vi "FipsAdjacent.vi"() -> (11 "Fips":i32[](array[numeric]))   [LabVIEW 2017] (continued)
IL\"\t17151\n\"Pope County, IL\"\t17151\t\"Saline County, IL\"\t17165\n\"Pope County, IL\"\t17151\t\"Williamson County, IL\"\t17199\n\"Pope County, IL\"\t17151\t\"Livingston County, KY\"\t21139\n\"Pulaski County, IL\"\t17153\t\"Alexander County, IL\"\t17003\n\"Pulaski County, IL\"\t17153\t\"Johnson County, IL\"\t17087\n\"Pulaski County, IL\"\t17153\t\"Massac County, IL\"\t17127\n\"Pulaski County, IL\"\t17153\t\"Pulaski County, IL\"\t17153\n\"Pulaski County, IL\"\t17153\t\"Union County, IL\"\t17181\n\"Pulaski County, IL\"\t17153\t\"Ballard County, KY\"\t21007\n\"Pulaski County, IL\"\t17153\t\"McCracken County, KY\"\t21145\n\"Putnam County, IL\"\t17155\t\"Bureau County, IL\"\t17011\n\"Putnam County, IL\"\t17155\t\"LaSalle County, IL\"\t17099\n\"Putnam County, IL\"\t17155\t\"Marshall County, IL\"\t17123\n\"Putnam County, IL\"\t17155\t\"Putnam County, IL\"\t17155\n\"Randolph County, IL\"\t17157\t\"Jackson County, IL\"\t17077\n\"Randolph County, IL\"\t17157\t\"Monroe County, IL\"\t17133\n\"Randolph County, IL\"\t17157\t\"Perry County, IL\"\t17145\n\"Randolph County, IL\"\t17157\t\"Randolph County, IL\"\t17157\n\"Randolph County, IL\"\t17157\t\"St. Clair County, IL\"\t17163\n\"Randolph County, IL\"\t17157\t\"Washington County, IL\"\t17189\n\"Randolph County, IL\"\t17157\t\"Perry County, MO\"\t29157\n\"Randolph County, IL\"\t17157\t\"Ste. Genevieve County, MO\"\t29186\n\"Richland County, IL\"\t17159\t\"Clay County, IL\"\t17025\n\"Richland County, IL\"\t17159\t\"Crawford County, IL\"\t17033\n\"Richland County, IL\"\t17159\t\"Edwards County, IL\"\t17047\n\"Richland County, IL\"\t17159\t\"Jasper County, IL\"\t17079\n\"Richland County, IL\"\t17159\t\"Lawrence County, IL\"\t17101\n\"Richland County, IL\"\t17159\t\"Richland County, IL\"\t17159\n\"Richland County, IL\"\t17159\t\"Wabash County, IL\"\t17185\n\"Richland County, IL\"\t17159\t\"Wayne County, IL\"\t17191\n\"Rock Island County, IL\"\t17161\t\"Henry County, IL\"\t17073\n\"Rock Island County, IL\"\t17161\t\"Mercer County, IL\"\t17131\n\"Rock Island County, IL\"\t17161\t\"Rock Island County, IL\"\t17161\n\"Rock Island County, IL\"\t17161\t\"Whiteside County, IL\"\t17195\n\"Rock Island County, IL\"\t17161\t\"Clinton County, IA\"\t19045\n\"Rock Island County, IL\"\t17161\t\"Louisa County, IA\"\t19115\n\"Rock Island County, IL\"\t17161\t\"Muscatine County, IA\"\t19139\n\"Rock Island County, IL\"\t17161\t\"Scott County, IA\"\t19163\n\"St. Clair County, IL\"\t17163\t\"Clinton County, IL\"\t17027\n\"St. Clair County, IL\"\t17163\t\"Madison County, IL\"\t17119\n\"St. Clair County, IL\"\t17163\t\"Monroe County, IL\"\t17133\n\"St. Clair County, IL\"\t17163\t\"Randolph County, IL\"\t17157\n\"St. Clair County, IL\"\t17163\t\"St. Clair County, IL\"\t17163\n\"St. Clair County, IL\"\t17163\t\"Washington County, IL\"\t17189\n\"St. Clair County, IL\"\t17163\t\"St. Louis County, MO\"\t29189\n\"St. Clair County, IL\"\t17163\t\"St. Louis city, MO\"\t29510\n\"Saline County, IL\"\t17165\t\"Franklin County, IL\"\t17055\n\"Saline County, IL\"\t17165\t\"Gallatin County, IL\"\t17059\n\"Saline County, IL\"\t17165\t\"Hamilton County, IL\"\t17065\n\"Saline County, IL\"\t17165\t\"Hardin County, IL\"\t17069\n\"Saline County, IL\"\t17165\t\"Johnson County, IL\"\t17087\n\"Saline County, IL\"\t17165\t\"Pope County, IL\"\t17151\n\"Saline County, IL\"\t17165\t\"Saline County, IL\"\t17165\n\"Saline County, IL\"\t17165\t\"Williamson County, IL\"\t17199\n\"Sangamon County, IL\"\t17167\t\"Cass County, IL\"\t17017\n\"Sangamon County, IL\"\t17167\t\"Christian County, IL\"\t17021\n\"Sangamon County, IL\"\t17167\t\"Logan County, IL\"\t17107\n\"Sangamon County, IL\"\t17167\t\"Macon County, IL\"\t17115\n\"Sangamon County, IL\"\t17167\t\"Macoupin County, IL\"\t17117\n\"Sangamon County, IL\"\t17167\t\"Menard County, IL\"\t17129\n\"Sangamon County, IL\"\t17167\t\"Montgomery County, IL\"\t17135\n\"Sangamon County, IL\"\t17167\t\"Morgan County, IL\"\t17137\n\"Sangamon County, IL\"\t17167\t\"Sangamon County, IL\"\t17167\n\"Schuyler County, IL\"\t17169\t\"Adams County, IL\"\t17001\n\"Schuyler County, IL\"\t17169\t\"Brown County, IL\"\t17009\n\"Schuyler County, IL\"\t17169\t\"Cass County, IL\"\t17017\n\"Schuyler County, IL\"\t17169\t\"Fulton County, IL\"\t17057\n\"Schuyler County, IL\"\t17169\t\"Hancock County, IL\"\t17067\n\"Schuyler County, IL\"\t17169\t\"McDonough County, IL\"\t17109\n\"Schuyler County, IL\"\t17169\t\"Mason County, IL\"\t17125\n\"Schuyler County, IL\"\t17169\t\"Schuyler County, IL\"\t17169\n\"Scott County, IL\"\t17171\t\"Greene County, IL\"\t17061\n\"Scott County, IL\"\t17171\t\"Morgan County, IL\"\t17137\n\"Scott County, IL\"\t17171\t\"Pike County, IL\"\t17149\n\"Scott County, IL\"\t17171\t\"Scott County, IL\"\t17171\n\"Shelby County, IL\"\t17173\t\"Christian County, IL\"\t17021\n\"Shelby County, IL\"\t17173\t\"Coles County, IL\"\t17029\n\"Shelby County, IL\"\t17173\t\"Cumberland County, IL\"\t17035\n\"Shelby County, IL\"\t17173\t\"Effingham County, IL\"\t17049\n\"Shelby County, IL\"\t17173\t\"Fayette County, IL\"\t17051\n\"Shelby County, IL\"\t17173\t\"Macon County, IL\"\t17115\n\"Shelby County, IL\"\t17173\t\"Montgomery County, IL\"\t17135\n\"Shelby County, IL\"\t17173\t\"Moultrie County, IL\"\t17139\n\"Shelby County, IL\"\t17173\t\"Shelby County, IL\"\t17173\n\"Stark County, IL\"\t17175\t\"Bureau County, IL\"\t17011\n\"Stark County, IL\"\t17175\t\"Henry County, IL\"\t17073\n\"Stark County, IL\"\t17175\t\"Knox County, IL\"\t17095\n\"Stark County, IL\"\t17175\t\"Marshall County, IL\"\t17123\n\"Stark County, IL\"\t17175\t\"Peoria County, IL\"\t17143\n\"Stark County, IL\"\t17175\t\"Stark County, IL\"\t17175\n\"Stephenson County, IL\"\t17177\t\"Carroll County, IL\"\t17015\n\"Stephenson County, IL\"\t17177\t\"Jo Daviess County, IL\"\t17085\n\"Stephenson County, IL\"\t17177\t\"Ogle County, IL\"\t17141\n\"Stephenson County, IL\"\t17177\t\"Stephenson County, IL\"\t17177\n\"Stephenson County, IL\"\t17177\t\"Winnebago County, IL\"\t17201\n\"Stephenson County, IL\"\t17177\t\"Green County, WI\"\t55045\n\"Stephenson County, IL\"\t17177\t\"Lafayette County, WI\"\t55065\n\"Tazewell County, IL\"\t17179\t\"Fulton County, IL\"\t17057\n\"Tazewell County, IL\"\t17179\t\"Logan County, IL\"\t17107\n\"Tazewell County, IL\"\t17179\t\"McLean County, IL\"\t17113\n\"Tazewell County, IL\"\t17179\t\"Mason County, IL\"\t17125\n\"Tazewell County, IL\"\t17179\t\"Peoria County, IL\"\t17143\n\"Tazewell County, IL\"\t17179\t\"Tazewell County, IL\"\t17179\n\"Tazewell County, IL\"\t17179\t\"Woodford County, IL\"\t17203\n\"Union County, IL\"\t17181\t\"Alexander County, IL\"\t17003\n\"Union County, IL\"\t17181\t\"Jackson County, IL\"\t17077\n\"Union County, IL\"\t17181\t\"Johnson County, IL\"\t17087\n\"Union County, IL\"\t17181\t\"Pulaski County, IL\"\t17153\n\"Union County, IL\"\t17181\t\"Union County, IL\"\t17181\n\"Union County, IL\"\t17181\t\"Williamson County, IL\"\t17199\n\"Union County, IL\"\t17181\t\"Cape Girardeau County, MO\"\t29031\n\"Union County, IL\"\t17181\t\"Perry County, MO\"\t29157\n\"Vermilion County, IL\"\t17183\t\"Champaign County, IL\"\t17019\n\"Vermilion County, IL\"\t17183\t\"Douglas County, IL\"\t17041\n\"Vermilion County, IL\"\t17183\t\"Edgar County, IL\"\t17045\n\"Vermilion County, IL\"\t17183\t\"Ford County, IL\"\t17053\n\"Vermilion County, IL\"\t17183\t\"Iroquois County, IL\"\t17075\n\"Vermilion County, IL\"\t17183\t\"Vermilion County, IL\"\t17183\n\"Vermilion County, IL\"\t17183\t\"Benton County, IN\"\t18007\n\"Vermilion County, IL\"\t17183\t\"Vermillion County, IN\"\t18165\n\"Vermilion County, IL\"\t17183\t\"Warren County, IN\"\t18171\n\"Wabash County, IL\"\t17185\t\"Edwards County, IL\"\t17047\n\"Wabash County, IL\"\t17185\t\"Lawrence County, IL\"\t17101\n\"Wabash County, IL\"\t17185\t\"Richland County, IL\"\t17159\n\"Wabash County, IL\"\t17185\t\"Wabash County, IL\"\t17185\n\"Wabash County, IL\"\t17185\t\"White County, IL\"\t17193\n\"Wabash County, IL\"\t17185\t\"Gibson County, IN\"\t18051\n\"Wabash County, IL\"\t17185\t\"Knox County, IN\"\t18083\n\"Warren County, IL\"\t17187\t\"Fulton County, IL\"\t17057\n\"Warren County, IL\"\t17187\t\"Henderson County, IL\"\t17071\n\"Warren County, IL\"\t17187\t\"Knox County, IL\"\t17095\n\"Warren County, IL\"\t17187\t\"McDonough County, IL\"\t17109\n\"Warren County, IL\"\t17187\t\"Mercer County, IL\"\t17131\n\"Warren County, IL\"\t17187\t\"Warren County, IL\"\t17187\n\"Washington County, IL\"\t17189\t\"Clinton County, IL\"\t17027\n\"Washington County, IL\"\t17189\t\"Jefferson County, IL\"\t17081\n\"Washington County, IL\"\t17189\t\"Marion County, IL\"\t17121\n\"Washington County, IL\"\t17189\t\"Perry County, IL\"\t17145\n\"Washington County, IL\"\t17189\t\"Randolph County, IL\"\t17157\n\"Washington County, IL\"\t17189\t\"St. Clair County, IL\"\t17163\n\"Washington County, IL\"\t17189\t\"Washington County, IL\"\t17189\n\"Wayne County, IL\"\t17191\t\"Clay County, IL\"\t17025\n\"Wayne County, IL\"\t17191\t\"Edwards County, IL\"\t17047\n\"Wayne County, IL\"\t17191\t\"Hamilton County, IL\"\t17065\n\"Wayne County, IL\"\t17191\t\"Jefferson County, IL\"\t17081\n\"Wayne County, IL\"\t17191\t\"Marion County, IL\"\t17121\n\"Wayne County, IL\"\t17191\t\"Richland County, IL\"\t17159\n\"Wayne County, IL\"\t17191\t\"Wayne County, IL\"\t17191\n\"Wayne County, IL\"\t17191\t\"White County, IL\"\t17193\n\"White County, IL\"\t17193\t\"Edwards County, IL\"\t17047\n\"White County, IL\"\t17193\t\"Gallatin County, IL\"\t17059\n\"White County, IL\"\t17193\t\"Hamilton County, IL\"\t17065\n\"White County, IL\"\t17193\t\"Wabash County, IL\"\t17185\n\"White County, IL\"\t17193\t\"Wayne County, IL\"\t17191\n\"White County, IL\"\t17193\t\"White County, IL\"\t17193\n\"White County, IL\"\t17193\t\"Gibson County, IN\"\t18051\n\"White County, IL\"\t17193\t\"Posey County, IN\"\t18129\n\"Whiteside County, IL\"\t17195\t\"Bureau County, IL\"\t17011\n\"Whiteside County, IL\"\t17195\t\"Carroll County, IL\"\t17015\n\"Whiteside County, IL\"\t17195\t\"Henry County, IL\"\t17073\n\"Whiteside County, IL\"\t17195\t\"Lee County, IL\"\t17103\n\"Whiteside County, IL\"\t17195\t\"Ogle County, IL\"\t17141\n\"Whiteside County, IL\"\t17195\t\"Rock Island County, IL\"\t17161\n\"Whiteside County, IL\"\t17195\t\"Whiteside County, IL\"\t17195\n\"Whiteside County, IL\"\t17195\t\"Clinton County, IA\"\t19045\n\"Will County, IL\"\t17197\t\"Cook County, IL\"\t17031\n\"Will County, IL\"\t17197\t\"DuPage County, IL\"\t17043\n\"Will County, IL\"\t17197\t\"Grundy County, IL\"\t17063\n\"Will County, IL\"\t17197\t\"Kankakee County, IL\"\t17091\n\"Will County, IL\"\t17197\t\"Kendall County, IL\"\t17093\n\"Will County, IL\"\t17197\t\"Will County, IL\"\t17197\n\"Will County, IL\"\t17197\t\"Lake County, IN\"\t18089\n\"Williamson County, IL\"\t17199\t\"Franklin County, IL\"\t17055\n\"Williamson County, IL\"\t17199\t\"Jackson County, IL\"\t17077\n\"Williamson County, IL\"\t17199\t\"Johnson County, IL\"\t17087\n\"Williamson County, IL\"\t17199\t\"Pope County, IL\"\t17151\n\"Williamson County, IL\"\t17199\t\"Saline County, IL\"\t17165\n\"Williamson County, IL\"\t17199\t\"Union County, IL\"\t17181\n\"Williamson County, IL\"\t17199\t\"Williamson County, IL\"\t17199\n\"Winnebago County, IL\"\t17201\t\"Boone County, IL\"\t17007\n\"Winnebago County, IL\"\t17201\t\"DeKalb County, IL\"\t17037\n\"Winnebago County, IL\"\t17201\t\"Ogle County, IL\"\t17141\n\"Winnebago County, IL\"\t17201\t\"Stephenson County, IL\"\t17177\n\"Winnebago County, IL\"\t17201\t\"Winnebago County, IL\"\t17201\n\"Winnebago County, IL\"\t17201\t\"Green County, WI\"\t55045\n\"Winnebago County, IL\"\t17201\t\"Rock County, WI\"\t55105\n\"Woodford County, IL\"\t17203\t\"LaSalle County, IL\"\t17099\n\"Woodford County, IL\"\t17203\t\"Livingston County, IL\"\t17105\n\"Woodford County, IL\"\t17203\t\"McLean County, IL\"\t17113\n\"Woodford County, IL\"\t17203\t\"Marshall County, IL\"\t17123\n\"Woodford County, IL\"\t17203\t\"Peoria County, IL\"\t17143\n\"Woodford County, IL\"\t17203\t\"Tazewell County, IL\"\t17179\n\"Woodford County, IL\"\t17203\t\"Woodford County, IL\"\t17203\n\"Adams County, IN\"\t18001\t\"Adams County, IN\"\t18001\n\"Adams County, IN\"\t18001\t\"Allen County, IN\"\t18003\n\"Adams County, IN\"\t18001\t\"Jay County, IN\"\t18075\n\"Adams County, IN\"\t18001\t\"Wells County, IN\"\t18179\n\"Adams County, IN\"\t18001\t\"Mercer County, OH\"\t39107\n\"Adams County, IN\"\t18001\t\"Van Wert County, OH\"\t39161\n\"Allen County, IN\"\t18003\t\"Adams County, IN\"\t18001\n\"Allen County, IN\"\t18003\t\"Allen County, IN\"\t18003\n\"Allen County, IN\"\t18003\t\"DeKalb County, IN\"\t18033\n\"Allen County, IN\"\t18003\t\"Huntington County, IN\"\t18069\n\"Allen County, IN\"\t18003\t\"Noble County, IN\"\t18113\n\"Allen County, IN\"\t18003\t\"Wells County, IN\"\t18179\n\"Allen County, IN\"\t18003\t\"Whitley County, IN\"\t18183\n\"Allen County, IN\"\t18003\t\"Defiance County, OH\"\t39039\n\"Allen County, IN\"\t18003\t\"Paulding County, OH\"\t39125\n\"Allen County, IN\"\t18003\t\"Van Wert County, OH\"\t39161\n\"Bartholomew County, IN\"\t18005\t\"Bartholomew County, IN\"\t18005\n\"Bartholomew County, IN\"\t18005\t\"Brown County, IN\"\t18013\n\"Bartholomew County, IN\"\t18005\t\"Decatur County, IN\"\t18031\n\"Bartholomew County, IN\"\t18005\t\"Jackson County, IN\"\t18071\n\"Bartholomew County, IN\"\t18005\t\"Jennings County, IN\"\t18079\n\"Bartholomew County, IN\"\t18005\t\"Johnson County, IN\"\t18081\n\"Bartholomew County, IN\"\t18005\t\"Shelby County, IN\"\t18145\n\"Benton County, IN\"\t18007\t\"Iroquois County, IL\"\t17075\n\"Benton County, IN\"\t18007\t\"Vermilion County, IL\"\t17183\n\"Benton County, IN\"\t18007\t\"Benton County, IN\"\t18007\n\"Benton County, IN\"\t18007\t\"Jasper County, IN\"\t18073\n\"Benton County, IN\"\t18007\t\"Newton County, IN\"\t18111\n\"Benton County, IN\"\t18007\t\"Tippecanoe County, IN\"\t18157\n\"Benton County, IN\"\t18007\t\"Warren County, IN\"\t18171\n\"Benton County, IN\"\t18007\t\"White County, IN\"\t18181\n\"Blackford County, IN\"\t18009\t\"Blackford County, IN\"\t18009\n\"Blackford County, IN\"\t18009\t\"Delaware County, IN\"\t18035\n\"Blackford County, IN\"\t18009\t\"Grant County, IN\"\t18053\n\"Blackford County, IN\"\t18009\t\"Jay County, IN\"\t18075\n\"Blackford County, IN\"\t18009\t\"Wells County, IN\"\t18179\n\"Boone County, IN\"\t18011\t\"Boone County, IN\"\t18011\n\"Boone County, IN\"\t18011\t\"Clinton County, IN\"\t18023\n\"Boone County, IN\"\t18011\t\"Hamilton County, IN\"\t18057\n\"Boone County, IN\"\t18011\t\"Hendricks County, IN\"\t18063\n\"Boone County, IN\"\t18011\t\"Marion County, IN\"\t18097\n\"Boone County, IN\"\t18011\t\"Montgomery County, IN\"\t18107\n\"Brown County, IN\"\t18013\t\"Bartholomew County, IN\"\t18005\n\"Brown County, IN\"\t18013\t\"Brown County, IN\"\t18013\n\"Brown County, IN\"\t18013\t\"Jackson County, IN\"\t18071\n\"Brown County, IN\"\t18013\t\"Johnson County, IN\"\t18081\n\"Brown County, IN\"\t18013\t\"Monroe County, IN\"\t18105\n\"Brown County, IN\"\t18013\t\"Morgan County, IN\"\t18109\n\"Carroll County, IN\"\t18015\t\"Carroll County, IN\"\t18015\n\"Carroll County, IN\"\t18015\t\"Cass County, IN\"\t18017\n\"Carroll County, IN\"\t18015\t\"Clinton County, IN\"\t18023\n\"Carroll County, IN\"\t18015\t\"Howard County, IN\"\t18067\n\"Carroll County, IN\"\t18015\t\"Tippecanoe County, IN\"\t18157\n\"Carroll County, IN\"\t18015\t\"White County, IN\"\t18181\n\"Cass County, IN\"\t18017\t\"Carroll County, IN\"\t18015\n\"Cass County, IN\"\t18017\t\"Cass County, IN\"\t18017\n\"Cass County, IN\"\t18017\t\"Fulton County, IN\"\t18049\n\"Cass County, IN\"\t18017\t\"Howard County, IN\"\t18067\n\"Cass County, IN\"\t18017\t\"Miami County, IN\"\t18103\n\"Cass County, IN\"\t18017\t\"Pulaski County, IN\"\t18131\n\"Cass County, IN\"\t18017\t\"White County, IN\"\t18181\n\"Clark County, IN\"\t18019\t\"Clark County, IN\"\t18019\n\"Clark County, IN\"\t18019\t\"Floyd County, IN\"\t18043\n\"Clark County, IN\"\t18019\t\"Jefferson County, IN\"\t18077\n\"Clark County, IN\"\t18019\t\"Scott County, IN\"\t18143\n\"Clark County, IN\"\t18019\t\"Washington County, IN\"\t18175\n\"Clark County, IN\"\t18019\t\"Jefferson County, KY\"\t21111\n\"Clark County, IN\"\t18019\t\"Oldham County, KY\"\t21185\n\"Clark County, IN\"\t18019\t\"Trimble County, KY\"\t21223\n\"Clay County, IN\"\t18021\t\"Clay County, IN\"\t18021\n\"Clay County, IN\"\t18021\t\"Greene County, IN\"\t18055\n\"Clay County, IN\"\t18021\t\"Owen County, IN\"\t18119\n\"Clay County, IN\"\t18021\t\"Parke County, IN\"\t18121\n\"Clay County, IN\"\t18021\t\"Putnam County, IN\"\t18133\n\"Clay County, IN\"\t18021\t\"Sullivan County, IN\"\t18153\n\"Clay County, IN\"\t18021\t\"Vigo County, IN\"\t18167\n\"Clinton County, IN\"\t18023\t\"Boone County, IN\"\t18011\n\"Clinton County, IN\"\t18023\t\"Carroll County, IN\"\t18015\n\"Clinton County, IN\"\t18023\t\"Clinton County, IN\"\t18023\n\"Clinton County, IN\"\t18023\t\"Hamilton County, IN\"\t18057\n\"Clinton County, IN\"\t18023\t\"Howard County, IN\"\t18067\n\"Clinton County, IN\"\t18023\t\"Montgomery County, IN\"\t18107\n\"Clinton County, IN\"\t18023\t\"Tippecanoe County, IN\"\t18157\n\"Clinton County, IN\"\t18023\t\"Tipton County, IN\"\t18159\n\"Crawford County, IN\"\t18025\t\"Crawford County, IN\"\t18025\n\"Crawford County, IN\"\t18025\t\"Dubois County, IN\"\t18037\n\"Crawford County, IN\"\t18025\t\"Harrison County, IN\"\t18061\n\"Crawford County, IN\"\t18025\t\"Orange County, IN\"\t18117\n\"Crawford County, IN\"\t18025\t\"Perry County, IN\"\t18123\n\"Crawford County, IN\"\t18025\t\"Washington County, IN\"\t18175\n\"Crawford County, IN\"\t18025\t\"Meade County, KY\"\t21163\n\"Daviess County, IN\"\t18027\t\"Daviess County, IN\"\t18027\n\"Daviess County, IN\"\t18027\t\"Dubois County, IN\"\t18037\n\"Daviess County, IN\"\t18027\t\"Greene County, IN\"\t18055\n\"Daviess County, IN\"\t18027\t\"Knox County, IN\"\t18083\n\"Daviess County, IN\"\t18027\t\"Martin County, IN\"\t18101\n\"Daviess County, IN\"\t18027\t\"Pike County, IN\"\t18125\n\"Dearborn County, IN\"\t18029\t\"Dearborn County, IN\"\t18029\n\"Dearborn County, IN\"\t18029\t\"Franklin County, IN\"\t18047\n\"Dearborn County, IN\"\t18029\t\"Ohio County, IN\"\t18115\n\"Dearborn County, IN\"\t18029\t\"Ripley County, IN\"\t18137\n\"Dearborn County, IN\"\t18029\t\"Boone County, KY\"\t21015\n\"Dearborn County, IN\"\t18029\t\"Butler County, OH\"\t39017\n\"Dearborn County, IN\"\t18029\t\"Hamilton County, OH\"\t39061\n\"Decatur County, IN\"\t18031\t\"Bartholomew County, IN\"\t18005\n\"Decatur County, IN\"\t18031\t\"Decatur County, IN\"\t18031\n\"Decatur County, IN\"\t18031\t\"Franklin County, IN\"\t18047\n\"Decatur County, IN\"\t18031\t\"Jennings County, IN\"\t18079\n\"Decatur County, IN\"\t18031\t\"Ripley County, IN\"\t18137\n\"Decatur County, IN\"\t18031\t\"Rush County, IN\"\t18139\n\"Decatur County, IN\"\t18031\t\"Shelby County, IN\"\t18145\n\"DeKalb County, IN\"\t18033\t\"Allen County, IN\"\t18003\n\"DeKalb County, IN\"\t18033\t\"DeKalb County, IN\"\t18033\n\"DeKalb County, IN\"\t18033\t\"LaGrange County, IN\"\t18087\n\"DeKalb County, IN\"\t18033\t\"Noble County, IN\"\t18113\n\"DeKalb County, IN\"\t18033\t\"Steuben County, IN\"\t18151\n\"DeKalb County, IN\"\t18033\t\"Defiance County, OH\"\t39039\n\"DeKalb County, IN\"\t18033\t\"Williams County, OH\"\t39171\n\"Delaware County, IN\"\t18035\t\"Blackford County, IN\"\t18009\n\"Delaware County, IN\"\t18035\t\"Delaware County, IN\"\t18035\n\"Delaware County, IN\"\t18035\t\"Grant County, IN\"\t18053\n\"Delaware County, IN\"\t18035\t\"Henry County, IN\"\t18065\n\"Delaware County, IN\"\t18035\t\"Jay County, IN\"\t18075\n\"Delaware County, IN\"\t18035\t\"Madison County, IN\"\t18095\n\"Delaware County, IN\"\t18035\t\"Randolph County, IN\"\t18135\n\"Dubois County, IN\"\t18037\t\"Crawford County, IN\"\t18025\n\"Dubois County, IN\"\t18037\t\"Daviess County, IN\"\t18027\n\"Dubois County, IN\"\t18037\t\"Dubois County, IN\"\t18037\n\"Dubois County, IN\"\t18037\t\"Martin County, IN\"\t18101\n\"Dubois County, IN\"\t18037\t\"Orange County, IN\"\t18117\n\"Dubois County, IN\"\t18037\t\"Perry County, IN\"\t18123\n\"Dubois County, IN\"\t18037\t\"Pike County, IN\"\t18125\n\"Dubois County, IN\"\t18037\t\"Spencer County, IN\"\t18147\n\"Dubois County, IN\"\t18037\t\"Warrick County, IN\"\t18173\n\"Elkhart County, IN\"\t18039\t\"Elkhart County, IN\"\t18039\n\"Elkhart County, IN\"\t18039\t\"Kosciusko County, IN\"\t18085\n\"Elkhart County, IN\"\t18039\t\"LaGrange County, IN\"\t18087\n\"Elkhart County, IN\"\t18039\t\"Marshall County, IN\"\t18099\n\"Elkhart County, IN\"\t18039\t\"Noble County, IN\"\t18113\n\"Elkhart County, IN\"\t18039\t\"St. Joseph County, IN\"\t18141\n\"Elkhart County, IN\"\t18039\t\"Cass County, MI\"\t26027\n\"Elkhart County, IN\"\t18039\t\"St. Joseph County, MI\"\t26149\n\"Fayette County, IN\"\t18041\t\"Fayette County, IN\"\t18041\n\"Fayette County, IN\"\t18041\t\"Franklin County, IN\"\t18047\n\"Fayette County, IN\"\t18041\t\"Henry County, IN\"\t18065\n\"Fayette County, IN\"\t18041\t\"Rush County, IN\"\t18139\n\"Fayette County, IN\"\t18041\t\"Union County, IN\"\t18161\n\"Fayette County, IN\"\t18041\t\"Wayne County, IN\"\t18177\n\"Floyd County, IN\"\t18043\t\"Clark County, IN\"\t18019\n\"Floyd County, IN\"\t18043\t\"Floyd County, IN\"\t18043\n\"Floyd County, IN\"\t18043\t\"Harrison County, IN\"\t18061\n\"Floyd County, IN\"\t18043\t\"Washington County, IN\"\t18175\n\"Floyd County, IN\"\t18043\t\"Jefferson County, KY\"\t21111\n\"Fountain County, IN\"\t18045\t\"Fountain County, IN\"\t18045\n\"Fountain County, IN\"\t18045\t\"Montgomery County, IN\"\t18107\n\"Fountain County, IN\"\t18045\t\"Parke County, IN\"\t18121\n\"Fountain County, IN\"\t18045\t\"Tippecanoe County, IN\"\t18157\n\"Fountain County, IN\"\t18045\t\"Vermillion County, IN\"\t18165\n\"Fountain County, IN\"\t18045\t\"Warren County, IN\"\t18171\n\"Franklin County, IN\"\t18047\t\"Dearborn County, IN\"\t18029\n\"Franklin County, IN\"\t18047\t\"Decatur County, IN\"\t18031\n\"Franklin County, IN\"\t18047\t\"Fayette County, IN\"\t18041\n\"Franklin County, IN\"\t18047\t\"Franklin County, IN\"\t18047\n\"Franklin County, IN\"\t18047\t\"Ripley County, IN\"\t18137\n\"Franklin County, IN\"\t18047\t\"Rush County, IN\"\t18139\n\"Franklin County, IN\"\t18047\t\"Union County, IN\"\t18161\n\"Franklin County, IN\"\t18047\t\"Butler County, OH\"\t39017\n\"Franklin County, IN\"\t18047\t\"Hamilton County, OH\"\t39061\n\"Fulton County, IN\"\t18049\t\"Cass County, IN\"\t18017\n\"Fulton County, IN\"\t18049\t\"Fulton County, IN\"\t18049\n\"Fulton County, IN\"\t18049\t\"Kosciusko County, IN\"\t18085\n\"Fulton County, IN\"\t18049\t\"Marshall County, IN\"\t18099\n\"Fulton County, IN\"\t18049\t\"Miami County, IN\"\t18103\n\"Fulton County, IN\"\t18049\t\"Pulaski County, IN\"\t18131\n\"Fulton County, IN\"\t18049\t\"Starke County, IN\"\t18149\n\"Fulton County, IN\"\t18049\t\"Wabash County, IN\"\t18169\n\"Gibson County, IN\"\t18051\t\"Wabash County, IL\"\t17185\n\"Gibson County, IN\"\t18051\t\"White County, IL\"\t17193\n\"Gibson County, IN\"\t18051\t\"Gibson County, IN\"\t18051\n\"Gibson County, IN\"\t18051\t\"Knox County, IN\"\t18083\n\"Gibson County, IN\"\t18051\t\"Pike County, IN\"\t18125\n\"Gibson County, IN\"\t18051\t\"Posey County, IN\"\t18129\n\"Gibson County, IN\"\t18051\t\"Vanderburgh County, IN\"\t18163\n\"Gibson County, IN\"\t18051\t\"Warrick County, IN\"\t18173\n\"Grant County, IN\"\t18053\t\"Blackford County, IN\"\t18009\n\"Grant County, IN\"\t18053\t\"Delaware County, IN\"\t18035\n\"Grant County, IN\"\t18053\t\"Grant County, IN\"\t18053\n\"Grant County, IN\"\t18053\t\"Howard County, IN\"\t18067\n\"Grant County, IN\"\t18053\t\"Huntington County, IN\"\t18069\n\"Grant County, IN\"\t18053\t\"Madison County, IN\"\t18095\n\"Grant County, IN\"\t18053\t\"Miami County, IN\"\t18103\n\"Grant County, IN\"\t18053\t\"Tipton County, IN\"\t18159\n\"Grant County, IN\"\t18053\t\"Wabash County, IN\"\t18169\n\"Grant County, IN\"\t18053\t\"Wells County, IN\"\t18179\n\"Greene County, IN\"\t18055\t\"Clay County, IN\"\t18021\n\"Greene County, IN\"\t18055\t\"Daviess County, IN\"\t18027\n\"Greene County, IN\"\t18055\t\"Greene County, IN\"\t18055\n\"Greene County, IN\"\t18055\t\"Knox County, IN\"\t18083\n\"Greene County, IN\"\t18055\t\"Lawrence County, IN\"\t18093\n\"Greene County, IN\"\t18055\t\"Martin County, IN\"\t18101\n\"Greene County, IN\"\t18055\t\"Monroe County, IN\"\t18105\n\"Greene County, IN\"\t18055\t\"Owen County, IN\"\t18119\n\"Greene County, IN\"\t18055\t\"Sullivan County, IN\"\t18153\n\"Hamilton County, IN\"\t18057\t\"Boone County, IN\"\t18011\n\"Hamilton County, IN\"\t18057\t\"Clinton County, IN\"\t18023\n\"Hamilton County, IN\"\t18057\t\"Hamilton County, IN\"\t18057\n\"Hamilton County, IN\"\t18057\t\"Hancock County, IN\"\t18059\n\"Hamilton County, IN\"\t18057\t\"Madison County, IN\"\t18095\n\"Hamilton County, IN\"\t18057\t\"Marion County, IN\"\t18097\n\"Hamilton County, IN\"\t18057\t\"Tipton County, IN\"\t18159\n\"Hancock County, IN\"\t18059\t\"Hamilton County, IN\"\t18057\n\"Hancock County, IN\"\t18059\t\"Hancock County, IN\"\t18059\n\"Hancock County, IN\"\t18059\t\"Henry County, IN\"\t18065\n\"Hancock County, IN\"\t18059\t\"Madison County, IN\"\t18095\n\"Hancock County, IN\"\t18059\t\"Marion County, IN\"\t18097\n\"Hancock County, IN\"\t18059\t\"Rush County, IN\"\t18139\n\"Hancock County, IN\"\t18059\t\"Shelby County, IN\"\t18145\n\"Harrison County, IN\"\t18061\t\"Crawford County, IN\"\t18025\n\"Harrison County, IN\"\t18061\t\"Floyd County, IN\"\t18043\n\"Harrison County, IN\"\t18061\t\"Harrison County, IN\"\t18061\n\"Harrison County, IN\"\t18061\t\"Washington County, IN\"\t18175\n\"Harrison County, IN\"\t18061\t\"Hardin County, KY\"\t21093\n\"Harrison County, IN\"\t18061\t\"Jefferson County, KY\"\t21111\n\"Harrison County, IN\"\t18061\t\"Meade County, KY\"\t21163\n\"Hendricks County, IN\"\t18063\t\"Boone County, IN\"\t18011\n\"Hendricks County, IN\"\t18063\t\"Hendricks County, IN\"\t18063\n\"Hendricks County, IN\"\t18063\t\"Marion County, IN\"\t18097\n\"Hendricks County, IN\"\t18063\t\"Montgomery County, IN\"\t18107\n\"Hendricks County, IN\"\t18063\t\"Morgan County, IN\"\t18109\n\"Hendricks County, IN\"\t18063\t\"Putnam County, IN\"\t18133\n\"Henry County, IN\"\t18065\t\"Delaware County, IN\"\t18035\n\"Henry County, IN\"\t18065\t\"Fayette County, IN\"\t18041\n\"Henry County, IN\"\t18065\t\"Hancock County, IN\"\t18059\n\"Henry County, IN\"\t18065\t\"Henry County, IN\"\t18065\n\"Henry County, IN\"\t18065\t\"Madison County, IN\"\t18095\n\"Henry County, IN\"\t18065\t\"Randolph County, IN\"\t18135\n\"Henry County, IN\"\t18065\t\"Rush County, IN\"\t18139\n\"Henry County, IN\"\t18065\t\"Wayne County, IN\"\t18177\n\"Howard County, IN\"\t18067\t\"Carroll County, IN\"\t18015\n\"Howard County, IN\"\t18067\t\"Cass County, IN\"\t18017\n\"Howard County, IN\"\t18067\t\"Clinton County, IN\"\t18023\n\"Howard County, IN\"\t18067\t\"Grant County, IN\"\t18053\n\"Howard County, IN\"\t18067\t\"Howard County, IN\"\t18067\n\"Howard County, IN\"\t18067\t\"Miami County, IN\"\t18103\n\"Howard County, IN\"\t18067\t\"Tipton County, IN\"\t18159\n\"Huntington County, IN\"\t18069\t\"Allen County, IN\"\t18003\n\"Huntington County, IN\"\t18069\t\"Grant County, IN\"\t18053\n\"Huntington County, IN\"\t18069\t\"Huntington County, IN\"\t18069\n\"Huntington County, IN\"\t18069\t\"Wabash County, IN\"\t18169\n\"Huntington County, IN\"\t18069\t\"Wells County, IN\"\t18179\n\"Huntington County, IN\"\t18069\t\"Whitley County, IN\"\t18183\n\"Jackson County, IN\"\t18071\t\"Bartholomew County, IN\"\t18005\n\"Jackson County, IN\"\t18071\t\"Brown County, IN\"\t18013\n\"Jackson County, IN\"\t18071\t\"Jackson County, IN\"\t18071\n\"Jackson County, IN\"\t18071\t\"Jennings County, IN\"\t18079\n\"Jackson County, IN\"\t18071\t\"Lawrence County, IN\"\t18093\n\"Jackson County, IN\"\t18071\t\"Monroe County, IN\"\t18105\n\"Jackson County, IN\"\t18071\t\"Scott County, IN\"\t18143\n\"Jackson County, IN\"\t18071\t\"Washington County, IN\"\t18175\n\"Jasper County, IN\"\t18073\t\"Benton County, IN\"\t18007\n\"Jasper County, IN\"\t18073\t\"Jasper County, IN\"\t18073\n\"Jasper County, IN\"\t18073\t\"Lake County, IN\"\t18089\n\"Jasper County, IN\"\t18073\t\"LaPorte County, IN\"\t18091\n\"Jasper County, IN\"\t18073\t\"Newton County, IN\"\t18111\n\"Jasper County, IN\"\t18073\t\"Porter County, IN\"\t18127\n\"Jasper County, IN\"\t18073\t\"Pulaski County, IN\"\t18131\n\"Jasper County, IN\"\t18073\t\"Starke County, IN\"\t18149\n\"Jasper County, IN\"\t18073\t\"White County, IN\"\t18181\n\"Jay County, IN\"\t18075\t\"Adams County, IN\"\t18001\n\"Jay County, IN\"\t18075\t\"Blackford County, IN\"\t18009\n\"Jay County, IN\"\t18075\t\"Delaware County, IN\"\t18035\n\"Jay County, IN\"\t18075\t\"Jay County, IN\"\t18075\n\"Jay County, IN\"\t18075\t\"Randolph County, IN\"\t18135\n\"Jay County, IN\"\t18075\t\"Wells County, IN\"\t18179\n\"Jay County, IN\"\t18075\t\"Darke County, OH\"\t39037\n\"Jay County, IN\"\t18075\t\"Mercer County, OH\"\t39107\n\"Jefferson County, IN\"\t18077\t\"Clark County, IN\"\t18019\n\"Jefferson County, IN\"\t18077\t\"Jefferson County, IN\"\t18077\n\"Jefferson County, IN\"\t18077\t\"Jennings County, IN\"\t18079\n\"Jefferson County, IN\"\t18077\t\"Ripley County, IN\"\t18137\n\"Jefferson County, IN\"\t18077\t\"Scott County, IN\"\t18143\n\"Jefferson County, IN\"\t18077\t\"Switzerland County, IN\"\t18155\n\"Jefferson County, IN\"\t18077\t\"Carroll County, KY\"\t21041\n\"Jefferson County, IN\"\t18077\t\"Trimble County, KY\"\t21223\n\"Jennings County, IN\"\t18079\t\"Bartholomew County, IN\"\t18005\n\"Jennings County, IN\"\t18079\t\"Decatur County, IN\"\t18031\n\"Jennings County, IN\"\t18079\t\"Jackson County, IN\"\t18071\n\"Jennings County, IN\"\t18079\t\"Jefferson County, IN\"\t18077\n\"Jennings County, IN\"\t18079\t\"Jennings County, IN\"\t18079\n\"Jennings County, IN\"\t18079\t\"Ripley County, IN\"\t18137\n\"Jennings County, IN\"\t18079\t\"Scott County, IN\"\t18143\n\"Johnson County, IN\"\t18081\t\"Bartholomew County, IN\"\t18005\n\"Johnson County, IN\"\t18081\t\"Brown County, IN\"\t18013\n\"Johnson County, IN\"\t18081\t\"Johnson County, IN\"\t18081\n\"Johnson County, IN\"\t18081\t\"Marion County, IN\"\t18097\n\"Johnson County, IN\"\t18081\t\"Morgan County, IN\"\t18109\n\"Johnson County, IN\"\t18081\t\"Shelby County, IN\"\t18145\n\"Knox County, IN\"\t18083\t\"Crawford County, IL\"\t17033\n\"Knox County, IN\"\t18083\t\"Lawrence County, IL\"\t17101\n\"Knox County, IN\"\t18083\t\"Wabash County, IL\"\t17185\n\"Knox County, IN\"\t18083\t\"Daviess County, IN\"\t18027\n\"Knox County, IN\"\t18083\t\"Gibson County, IN\"\t18051\n\"Knox County, IN\"\t18083\t\"Greene County, IN\"\t18055\n\"Knox County, IN\"\t18083\t\"Knox County, IN\"\t18083\n\"Knox County, IN\"\t18083\t\"Pike County, IN\"\t18125\n\"Knox County, IN\"\t18083\t\"Sullivan County, IN\"\t18153\n\"Kosciusko County, IN\"\t18085\t\"Elkhart County, IN\"\t18039\n\"Kosciusko County, IN\"\t18085\t\"Fulton County, IN\"\t18049\n\"Kosciusko County, IN\"\t18085\t\"Kosciusko County, IN\"\t18085\n\"Kosciusko County, IN\"\t18085\t\"Marshall County, IN\"\t18099\n\"Kosciusko County, IN\"\t18085\t\"Noble County, IN\"\t18113\n\"Kosciusko County, IN\"\t18085\t\"Wabash County, IN\"\t18169\n\"Kosciusko County, IN\"\t18085\t\"Whitley County, IN\"\t18183\n\"LaGrange County, IN\"\t18087\t\"DeKalb County, IN\"\t18033\n\"LaGrange County, IN\"\t18087\t\"Elkhart County, IN\"\t18039\n\"LaGrange County, IN\"\t18087\t\"LaGrange County, IN\"\t18087\n\"LaGrange County, IN\"\t18087\t\"Noble County, IN\"\t18113\n\"LaGrange County, IN\"\t18087\t\"Steuben County, IN\"\t18151\n\"LaGrange County, IN\"\t18087\t\"Branch County, MI\"\t26023\n\"LaGrange County, IN\"\t18087\t\"St. Joseph County, MI\"\t26149\n\"Lake County, IN\"\t18089\t\"Cook County, IL\"\t17031\n\"Lake County, IN\"\t18089\t\"Kankakee County, IL\"\t17091\n\"Lake County, IN\"\t18089\t\"Will County, IL\"\t17197\n\"Lake County, IN\"\t18089\t\"Jasper County, IN\"\t18073\n\"Lake County, IN\"\t18089\t\"Lake County, IN\"\t18089\n\"Lake County, IN\"\t18089\t\"Newton County, IN\"\t18111\n\"Lake County, IN\"\t18089\t\"Porter County, IN\"\t18127\n\"LaPorte County, IN\"\t18091\t\"Jasper County, IN\"\t18073\n\"LaPorte County, IN\"\t18091\t\"LaPorte County, IN\"\t18091\n\"LaPorte County, IN\"\t18091\t\"Porter County, IN\"\t18127\n\"LaPorte County, IN\"\t18091\t\"St. Joseph County, IN\"\t18141\n\"LaPorte County, IN\"\t18091\t\"Starke County, IN\"\t18149\n\"LaPorte County, IN\"\t18091\t\"Berrien County, MI\"\t26021\n\"Lawrence County, IN\"\t18093\t\"Greene County, IN\"\t18055\n\"Lawrence County, IN\"\t18093\t\"Jackson County, IN\"\t18071\n\"Lawrence County, IN\"\t18093\t\"Lawrence County, IN\"\t18093\n\"Lawrence County, IN\"\t18093\t\"Martin County, IN\"\t18101\n\"Lawrence County, IN\"\t18093\t\"Monroe County, IN\"\t18105\n\"Lawrence County, IN\"\t18093\t\"Orange County, IN\"\t18117\n\"Lawrence County, IN\"\t18093\t\"Washington County, IN\"\t18175\n\"Madison County, IN\"\t18095\t\"Delaware County, IN\"\t18035\n\"Madison County, IN\"\t18095\t\"Grant County, IN\"\t18053\n\"Madison County, IN\"\t18095\t\"Hamilton County, IN\"\t18057\n\"Madison County, IN\"\t18095\t\"Hancock County, IN\"\t18059\n\"Madison County, IN\"\t18095\t\"Henry County, IN\"\t18065\n\"Madison County, IN\"\t18095\t\"Madison County, IN\"\t18095\n\"Madison County, IN\"\t18095\t\"Tipton County, IN\"\t18159\n\"Marion County, IN\"\t18097\t\"Boone County, IN\"\t18011\n\"Marion County, IN\"\t18097\t\"Hamilton County, IN\"\t18057\n\"Marion County, IN\"\t18097\t\"Hancock County, IN\"\t18059\n\"Marion County, IN\"\t18097\t\"Hendricks County, IN\"\t18063\n\"Marion County, IN\"\t18097\t\"Johnson County, IN\"\t18081\n\"Marion County, IN\"\t18097\t\"Marion County, IN\"\t18097\n\"Marion County, IN\"\t18097\t\"Morgan County, IN\"\t18109\n\"Marion County, IN\"\t18097\t\"Shelby County, IN\"\t18145\n\"Marshall County, IN\"\t18099\t\"Elkhart County, IN\"\t18039\n\"Marshall County, IN\"\t18099\t\"Fulton County, IN\"\t18049\n\"Marshall County, IN\"\t18099\t\"Kosciusko County, IN\"\t18085\n\"Marshall County, IN\"\t18099\t\"Marshall County, IN\"\t18099\n\"Marshall County, IN\"\t18099\t\"Pulaski County, IN\"\t18131\n\"Marshall County, IN\"\t18099\t\"St. Joseph County, IN\"\t18141\n\"Marshall County, IN\"\t18099\t\"Starke County, IN\"\t18149\n\"Martin County, IN\"\t18101\t\"Daviess County, IN\"\t18027\n\"Martin County, IN\"\t18101\t\"Dubois County, IN\"\t18037\n\"Martin County, IN\"\t18101\t\"Greene County, IN\"\t18055\n\"Martin County, IN\"\t18101\t\"Lawrence County, IN\"\t18093\n\"Martin County, IN\"\t18101\t\"Martin County, IN\"\t18101\n\"Martin County, IN\"\t18101\t\"Orange County, IN\"\t18117\n\"Miami County, IN\"\t18103\t\"Cass County, IN\"\t18017\n\"Miami County, IN\"\t18103\t\"Fulton County, IN\"\t18049\n\"Miami County, IN\"\t18103\t\"Grant County, IN\"\t18053\n\"Miami County, IN\"\t18103\t\"Howard County, IN\"\t18067\n\"Miami County, IN\"\t18103\t\"Miami County, IN\"\t18103\n\"Miami County, IN\"\t18103\t\"Wabash County, IN\"\t18169\n\"Monroe County, IN\"\t18105\t\"Brown County, IN\"\t18013\n\"Monroe County, IN\"\t18105\t\"Greene County, IN\"\t18055\n\"Monroe County, IN\"\t18105\t\"Jackson County, IN\"\t18071\n\"Monroe County, IN\"\t18105\t\"Lawrence County, IN\"\t18093\n\"Monroe County, IN\"\t18105\t\"Monroe County, IN\"\t18105\n\"Monroe County, IN\"\t18105\t\"Morgan County, IN\"\t18109\n\"Monroe County, IN\"\t18105\t\"Owen County, IN\"\t18119\n\"Montgomery County, IN\"\t18107\t\"Boone County, IN\"\t18011\n\"Montgomery County, IN\"\t18107\t\"Clinton County, IN\"\t18023\n\"Montgomery County, IN\"\t18107\t\"Fountain County, IN\"\t18045\n\"Montgomery County, IN\"\t18107\t\"Hendricks County, IN\"\t18063\n\"Montgomery County, IN\"\t18107\t\"Montgomery County, IN\"\t18107\n\"Montgomery County, IN\"\t18107\t\"Parke County, IN\"\t18121\n\"Montgomery County, IN\"\t18107\t\"Putnam County, IN\"\t18133\n\"Montgomery County, IN\"\t18107\t\"Tippecanoe County, IN\"\t18157\n\"Morgan County, IN\"\t18109\t\"Brown County, IN\"\t18013\n\"Morgan County, IN\"\t18109\t\"Hendricks County, IN\"\t18063\n\"Morgan County, IN\"\t18109\t\"Johnson County, IN\"\t18081\n\"Morgan County, IN\"\t18109\t\"Marion County, IN\"\t18097\n\"Morgan County, IN\"\t18109\t\"Monroe County, IN\"\t18105\n\"Morgan County, IN\"\t18109\t\"Morgan County, IN\"\t18109\n\"Morgan County, IN\"\t18109\t\"Owen County, IN\"\t18119\n\"Morgan County, IN\"\t18109\t\"Putnam County, IN\"\t18133\n\"Newton County, IN\"\t18111\t\"Iroquois County, IL\"\t17075\n\"Newton County, IN\"\t18111\t\"Kankakee County, IL\"\t17091\n\"Newton County, IN\"\t18111\t\"Benton County, IN\"\t18007\n\"Newton County, IN\"\t18111\t\"Jasper County, IN\"\t18073\n\"Newton County, IN\"\t18111\t\"Lake County, IN\"\t18089\n\"Newton County, IN\"\t18111\t\"Newton County, IN\"\t18111\n\"Noble County, IN\"\t18113\t\"Allen County, IN\"\t18003\n\"Noble County, IN\"\t18113\t\"DeKalb County, IN\"\t18033\n\"Noble County, IN\"\t18113\t\"Elkhart County, IN\"\t18039\n\"Noble County, IN\"\t18113\t\"Kosciusko County, IN\"\t18085\n\"Noble County, IN\"\t18113\t\"LaGrange County, IN\"\t18087\n\"Noble County, IN\"\t18113\t\"Noble County, IN\"\t18113\n\"Noble County, IN\"\t18113\t\"Steuben County, IN\"\t18151\n\"Noble County, IN\"\t18113\t\"Whitley County, IN\"\t18183\n\"Ohio County, IN\"\t18115\t\"Dearborn County, IN\"\t18029\n\"Ohio County, IN\"\t18115\t\"Ohio County, IN\"\t18115\n\"Ohio County, IN\"\t18115\t\"Ripley County, IN\"\t18137\n\"Ohio County, IN\"\t18115\t\"Switzerland County, IN\"\t18155\n\"Ohio County, IN\"\t18115\t\"Boone County, KY\"\t21015\n\"Orange County, IN\"\t18117\t\"Crawford County, IN\"\t18025\n\"Orange County, IN\"\t18117\t\"Dubois County, IN\"\t18037\n\"Orange County, IN\"\t18117\t\"Lawrence County, IN\"\t18093\n\"Orange County, IN\"\t18117\t\"Martin County, IN\"\t18101\n\"Orange County, IN\"\t18117\t\"Orange County, IN\"\t18117\n\"Orange County, IN\"\t18117\t\"Washington County, IN\"\t18175\n\"Owen County, IN\"\t18119\t\"Clay County, IN\"\t18021\n\"Owen County, IN\"\t18119\t\"Greene County, IN\"\t18055\n\"Owen County, IN\"\t18119\t\"Monroe County, IN\"\t18105\n\"Owen County, IN\"\t18119\t\"Morgan County, IN\"\t18109\n\"Owen County, IN\"\t18119\t\"Owen County, IN\"\t18119\n\"Owen County, IN\"\t18119\t\"Putnam County, IN\"\t18133\n\"Parke County, IN\"\t18121\t\"Clay County, IN\"\t18021\n\"Parke County, IN\"\t18121\t\"Fountain County, IN\"\t18045\n\"Parke County, IN\"\t18121\t\"Montgomery County, IN\"\t18107\n\"Parke County, IN\"\t18121\t\"Parke County, IN\"\t18121\n\"Parke County, IN\"\t18121\t\"Putnam County, IN\"\t18133\n\"Parke County, IN\"\t18121\t\"Vermillion County, IN\"\t18165\n\"Parke County, IN\"\t18121\t\"Vigo County, IN\"\t18167\n\"Perry County, IN\"\t18123\t\"Crawford County, IN\"\t18025\n\"Perry County, IN\"\t18123\t\"Dubois County, IN\"\t18037\n\"Perry County, IN\"\t18123\t\"Perry County, IN\"\t18123\n\"Perry County, IN\"\t18123\t\"Spencer County, IN\"\t18147\n\"Perry County, IN\"\t18123\t\"Breckinridge County, KY\"\t21027\n\"Perry County, IN\"\t18123\t\"Hancock County, KY\"\t21091\n\"Perry County, IN\"\t18123\t\"Meade County, KY\"\t21163\n\"Pike County, IN\"\t18125\t\"Daviess County, IN\"\t18027\n\"Pike County, IN\"\t18125\t\"Dubois County, IN\"\t18037\n\"Pike County, IN\"\t18125\t\"Gibson County, IN\"\t18051\n\"Pike County, IN\"\t18125\t\"Knox County, IN\"\t18083\n\"Pike County, IN\"\t18125\t\"Pike County, IN\"\t18125\n\"Pike County, IN\"\t18125\t\"Warrick County, IN\"\t18173\n\"Porter County, IN\"\t18127\t\"Cook County, IL\"\t17031\n\"Porter County, IN\"\t18127\t\"Jasper County, IN\"\t18073\n\"Porter County, IN\"\t18127\t\"Lake County, IN\"\t18089\n\"Porter County, IN\"\t18127\t\"LaPorte County, IN\"\t18091\n\"Porter County, IN\"\t18127\t\"Porter County, IN\"\t18127\n\"Porter County, IN\"\t18127\t\"Starke County, IN\"\t18149\n\"Porter County, IN\"\t18127\t\"Berrien County, MI\"\t26021\n\"Posey County, IN\"\t18129\t\"Gallatin County, IL\"\t17059\n\"Posey County, IN\"\t18129\t\"White County, IL\"\t17193\n\"Posey County, IN\"\t18129\t\"Gibson County, IN\"\t18051\n\"Posey County, IN\"\t18129\t
